vi "TestThor.vi"() -> ()   [LabVIEW 2019, in "Temperhum.Thorlabs.lvclass"]
uses:
  Temperhum.Thorlabs.lvclass
  drivers/TLTSP/TLTSP.lvlib
panel:
  out "error out":errorcluster
  out "TH1 Value":dbl caption="Temperature Value"
  out "Humidity":dbl
  out "Temperature":dbl
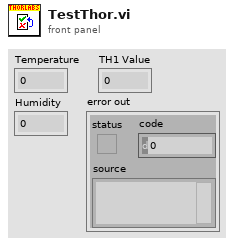
[diagram p1: front panel]
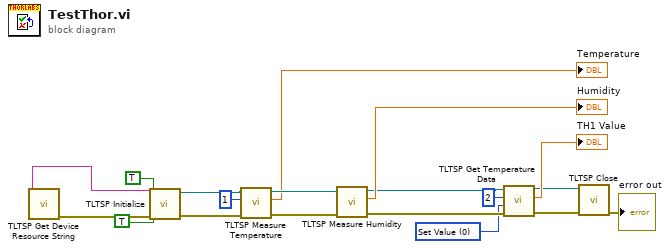
[diagram p0: block diagram]
diagram:
  w1 = i16 0 items=["Set Value", "Minimum value", "Maximum value"] ("Attribute (Set Value)")
  n1 = call "TLTSP Get Device Resource String.vi"() -> ("error out"=w8:errorcluster, "Resource Name"=w9:string)  [unwired: 9 in, 1 out]
  n2 = call "TLTSP Initialize.vi"("error in (no error)"=w8, "Reset Device (Reset Device)"=TRUE, "ID Query (Do Query)"=TRUE, "resource name"=w9) -> ("error out"=w7:errorcluster, "instrument handle out"=w10:refnum<visa-resource-name>)  [unwired: 6 in]
  n3 = call "TLTSP Measure Temperature.vi"("error in (no error)"=w7, "Channel (1)"=u16 1, "instrument handle"=w10) -> ("error out"=w6:errorcluster, "Temperature"=→"Temperature":dbl, "instrument handle out"=w19:refnum<visa-resource-name>)  [unwired: 6 in]
  n4 = call "TLTSP Measure Humidity.vi"("error in (no error)"=w6, "instrument handle"=w19) -> ("error out"=w5:errorcluster, "Humidity"=→"Humidity":dbl, "instrument handle out"=w16:refnum<visa-resource-name>)  [unwired: 7 in]
  n5 = call "TLTSP Get Temperature Data.vi"("error in (no error)"=w5, "Attribute (Set Value)"=w1, "Channel (1)"=u16 2, "instrument handle"=w16) -> ("error out"=w4:errorcluster, "Temperature Value"=→"TH1 Value":dbl, "instrument handle out"=w13:refnum<visa-resource-name>)  [unwired: 5 in]
  n6 = call "TLTSP Close.vi"("error in (no error)"=w4, "instrument handle"=w13) -> ("error out"=→"error out":errorcluster)  [unwired: 9 in]
